vi "Method_Const.vi"(4 "Value":u8, 5 "Input A":refnum<class "Abs_U8 Integer.lvclass">) -> (1 "Result":T1)   [LabVIEW 2021, in "Add_U8.lvclass"]
uses:
  Add_U8.lvclass
  Abs_Types/U8 Integer/Abs_U8 Integer.lvclass
  Abs_Type.ctl
  C:/TSA/LV_Abstract/Source/Functions/Support/Function/Two Terminal/U8/AbsFunc_Two Term_U8.lvclass
  C:/Program Files (x86)/National Instruments/LabVIEW 2021/vi.lib/TSA/Abstract Data Classes/Abs_Types/U8 Integer/Abs_U8 Integer.lvclass
  Support/Function/Two Terminal/U8/AbsFunc_Two Term_U8.lvclass/AbsFunc_Two Term_U8.ctl
  Support/Function/Two Terminal/U8/Properties/Write Numeric A.vi
  Support/Function/Two Terminal/U8/Properties/Write Numeric B.vi
  Constants/Support/U8/Const_U8.lvclass
  C:/Program Files (x86)/National Instruments/LabVIEW 2021/vi.lib/TSA/Abstract Data Classes/Abs_Types/Numeric/Abs_Numeric.lvclass
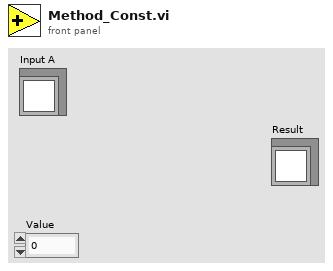
[diagram p1: front panel]
types:
  T1 = typedef "Add_U8.lvclass/Abs_Type.ctl" = refnum<class "Abs_U8 Integer.lvclass">
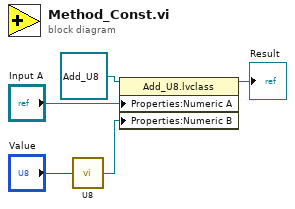
[diagram p0: block diagram]
diagram:
  n1 = call "U8.vi"("Value"="Value") -> ("Constant"=w2:refnum<class "Const_U8.lvclass">)  [unwired: 4 in]
  n2 = property class="Add_U8.lvclass"(reference=refnum<class "Add_U8.lvclass"> refnum ("Functions.lvlib:Numeric.lvlib:Add_SGL.lvclass"), "Properties:Numeric A"="Input A", "Properties:Numeric B"=w2) -> (reference out=→"Result":refnum<class "Add_U8.lvclass">)  [unwired: 1 in, 1 out]
